vi "CTRE_ServoBlock_All.vi"   [LabVIEW 2016]
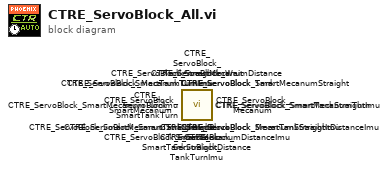
[diagram p0: block diagram]
diagram:
  n1 = call <vilib>:"CTRE_ServoBlock_SmartTank.vi"() -> ()  [unwired: 11 in, 1 out]
  n2 = call <vilib>:"CTRE_ServoBlock_Tank.vi"() -> ()  [unwired: 12 in]
  n3 = call <vilib>:"CTRE_ServoBlock_SmartMecanum.vi"() -> ()  [unwired: 11 in, 1 out]
  n4 = call <vilib>:"CTRE_ServoBlock_Mecanum.vi"() -> ()  [unwired: 11 in, 1 out]
  n5 = call <vilib>:"CTRE_ServoBlock_Wait.vi"() -> ()  [unwired: 12 in]
  n6 = call <vilib>:"CTRE_ServoBlock_MecanumTurnImu.vi"() -> ()  [unwired: 10 in, 2 out]
  n7 = call <vilib>:"CTRE_ServoBlock_MecanumStraightImu.vi"() -> ()  [unwired: 11 in, 1 out]
  n8 = call <vilib>:"CTRE_ServoBlock_TankTurnImu.vi"() -> ()  [unwired: 10 in, 2 out]
  n9 = call <vilib>:"CTRE_ServoBlock_TankStraightImu.vi"() -> ()  [unwired: 11 in, 1 out]
  n10 = call <vilib>:"CTRE_ServoBlock_SmartMecanumTurnImu.vi"() -> ()  [unwired: 10 in, 2 out]
  n11 = call <vilib>:"CTRE_ServoBlock_SmartMecanumTurn.vi"() -> ()  [unwired: 10 in, 2 out]
  n12 = call <vilib>:"CTRE_ServoBlock_SmartMecanumStraightImu.vi"() -> ()  [unwired: 11 in, 1 out]
  n13 = call <vilib>:"CTRE_ServoBlock_SmartMecanumStraight.vi"() -> ()  [unwired: 11 in, 1 out]
  n14 = call <vilib>:"CTRE_ServoBlock_SmartMecanumDistanceImu.vi"() -> ()  [unwired: 10 in, 2 out]
  n15 = call <vilib>:"CTRE_ServoBlock_SmartMecanumDistance.vi"() -> ()  [unwired: 10 in, 2 out]
  n16 = call <vilib>:"CTRE_ServoBlock_SmartTankTurnImu.vi"() -> ()  [unwired: 10 in, 2 out]
  n17 = call <vilib>:"CTRE_ServoBlock_SmartTankTurn.vi"() -> ()  [unwired: 10 in, 2 out]
  n18 = call <vilib>:"CTRE_ServoBlock_SmartTankStraightImu.vi"() -> ()  [unwired: 11 in, 1 out]
  n19 = call <vilib>:"CTRE_ServoBlock_SmartTankStraightDistanceImu.vi"() -> ()  [unwired: 10 in, 2 out]
  n20 = call <vilib>:"CTRE_ServoBlock_SmartTankStraightDistance.vi"() -> ()  [unwired: 10 in, 2 out]
  n21 = call <vilib>:"CTRE_ServoBlock_SmartTankStraight.vi"() -> ()  [unwired: 11 in, 1 out]
